vi "Variable global funcional.vi"(10 "Action":enum16{"Get", "Set"}(ring), 11 "New value":bool=TRUE) -> (3 "Output value":bool)   [LabVIEW 2020]
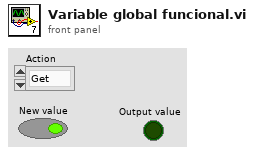
[diagram p1: front panel]
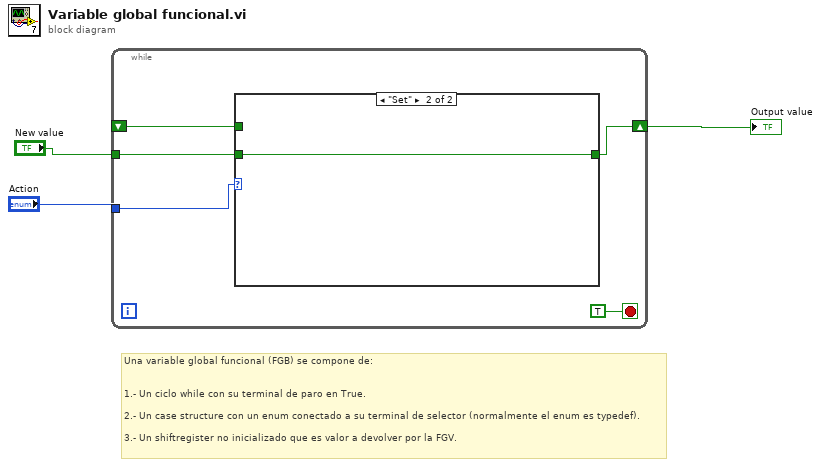
[diagram p0: block diagram]
diagram:
  # "Una variable global funcional (FGB) se compone de:\n\n\n1.- Un ciclo while con su terminal de paro en True.\n\n2.- Un case structure con un enum conectado a su terminal de selector (normalmente el enum es typedef).\n\n3.- Un shiftregister no inicializado que es valor a devolver por la FGV."
  n1 = while {
    tunnel: "Action" -> [w7]
    tunnel: "New value" -> [w6]
    shift-right: [w5] -> w1
    shift-left: _ -> [w4]
    stop <- TRUE stop-if-true
    n2 = case shown="\"Set\"" w7 {
      tunnel: [w9 w10] -> w5
      tunnel: w6 -> [_ w10]
      tunnel: w4 -> [w9 _]
      frame "Get", Default {
      }
      frame "Set" {
      }
    }
  }
  "Output value" <- w1
